vi "6.2.DHT22 Temp-Humidity Sensor -ThingSpeak.vi"   [LabVIEW 2014]
uses:
  <vilib>/Aledyne-TSXperts/Arduino Compatible Compiler for LabVIEW/addons/QwaveSys_ESP8266/QwaveSys_ESP8266.lvlib
  <vilib>/Aledyne-TSXperts/Arduino Compatible Compiler for LabVIEW/addons/QwaveSys_Interface/QwaveSys_Interface.lvlib
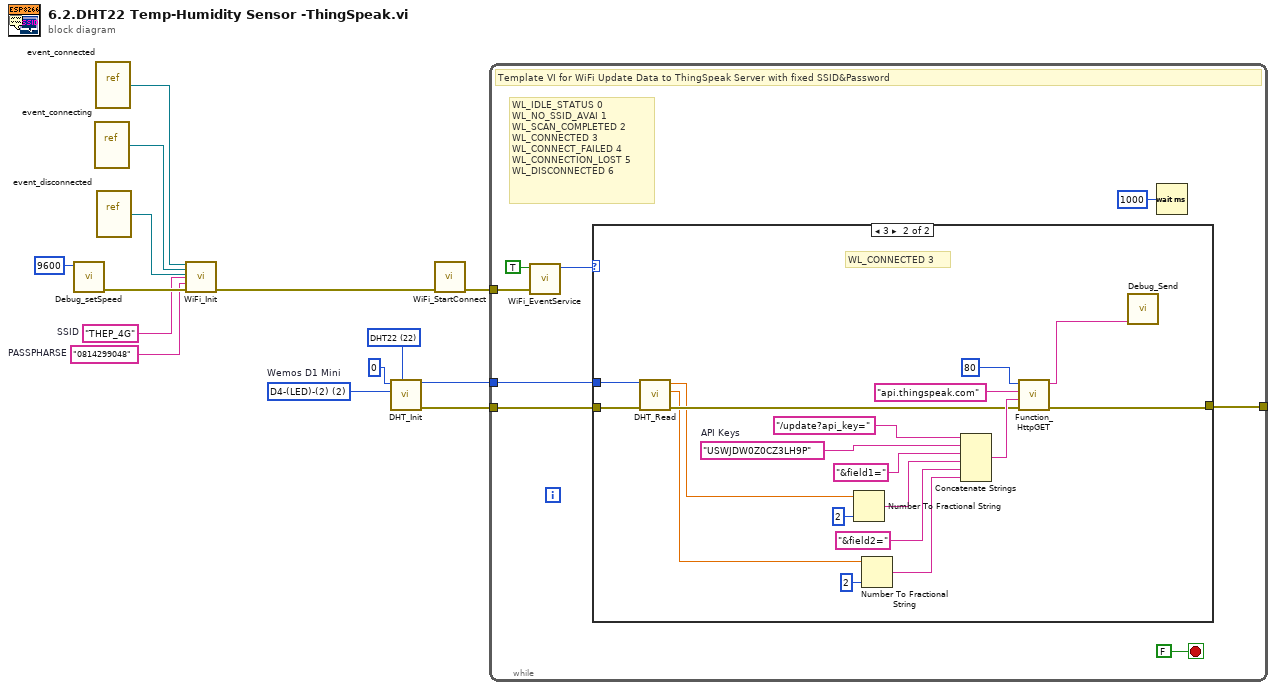
[diagram p0: block diagram]
diagram:
  w3 = u8 2 items=["D0-(16)"=16, "D1-SCL(5)"=5, "D2-SDA(4)"=4, "D3-(0)"=0, "D4-(LED)-(2)"=2, "D5-SCK(14)"=14, "D6-MISO(12)"=12, "D7-MOSI(13)"=13, "D8-SS(15)"=15, "TX(3)"=3, "RX(1)"=1, "ADC0,(17)"=17]  # Wemos D1 Mini
  w5 = u16 22 items=["DHT11"=11, "DHT21"=21, "DHT22"=22] ("Type")
  w7 = "0814299048"  # PASSPHARSE
  w8 = "THEP_4G"  # SSID
  n1 = call <vilib>:"Debug_setSpeed.vi"("Speed"=u32 9600) -> ("error out"=w10:errorcluster)  [unwired: 10 in]
  n2 = vi-ref "event_connecting.vi"() -> (w13:refnum<vi>)
  n3 = vi-ref "event_connected.vi"() -> (w12:refnum<vi>)
  n4 = vi-ref "event_disconnected.vi"() -> (w11:refnum<vi>)
  n5 = call <vilib>:"WiFi_Init.vi"("connected"=w12, "connecting"=w13, "disconnected"=w11, "SSID"=w8, "PASSPHARSE"=w7, "error in (no error)"=w10) -> ("error out"=w6:errorcluster)  [unwired: 9 in]
  n6 = call <vilib>:"DHT_Init.vi"("Type"=w5, "PIN"=w3, "Interface (0-4)"=u8 0) -> ("error out"=w2:errorcluster, "Instance"=w1:u8)  [unwired: 7 in]
  n7 = call <vilib>:"WiFi_StartConnect.vi"("error in (no error)"=w6) -> ("error out"=w14:errorcluster)  [unwired: 10 in]
  n8 = while {
    tunnel: w14 -> [w21]
    tunnel: [w17] -> _
    tunnel: w2 -> [w16]
    tunnel: w1 -> [w15]
    stop <- FALSE stop-if-true
    # "WL_IDLE_STATUS\t0\nWL_NO_SSID_AVAI\t1\nWL_SCAN_COMPLETED\t2\nWL_CONNECTED\t3\nWL_CONNECT_FAILED\t4\nWL_CONNECTION_LOST\t5\nWL_DISCONNECTED\t6"
    # "Template VI for WiFi Update Data to ThingSpeak Server with fixed SSID&Password"
    n9 = call <vilib>:"WiFi_EventService.vi"("error in (no error)"=w21, "wait for connected (True)"=TRUE) -> ("Status"=w18:u16)  [unwired: 8 in, 1 out]
    n10 = case shown="3" w18 {
      tunnel: [w23 w24] -> w17
      tunnel: w16 -> [w23 w29]
      tunnel: w15 -> [_ w27]
      frame 0, Default {
        # "DISCONNECTED or default status"
      }
      frame 3 {
        w32 = "USWJDW0Z0CZ3LH9P"  # API Keys
        # "WL_CONNECTED\t3"
        n11 = call <vilib>:"DHT_Read.vi"("Instance"=w27, "error in (no error)"=w29) -> ("error out"=w28:errorcluster, "Celsius"=w26:dbl, "Humidity"=w25:dbl)  [unwired: 4 in, 3 out]
        n12 = Number To Fractional String(number=w25, precision (6)=i16 2) -> (F-format string=w36:string)  [unwired: 2 in]
        n13 = Number To Fractional String(number=w26, precision (6)=i16 2) -> (F-format string=w39:string)  [unwired: 2 in]
        n14 = Concatenate Strings("/update?api_key=", w32, "&field1=", w36, "&field2=", w39) -> (w33:string)
        n15 = call <vilib>:"Function_HttpGET.vi"("error in (no error)"=w28, "URI"=w33, "Host"="api.thingspeak.com", "Port"=i8 80) -> ("error out"=w24:errorcluster, "Results"=w30:string)  [unwired: 6 in]
        n16 = call <vilib>:"Debug_Send.vi"("DATA"=w30) -> ()  [unwired: 11 in]
      }
    }
    n17 = Wait (ms)(milliseconds to wait=u32 1000) -> ()  [unwired: 1 out]
  }
